vi "Error MSG VicErrorParsing.vi"(11 "WrrmsgIn":string) -> (3 "MsgOut":string[][](array[string]))   [LabVIEW 2019]
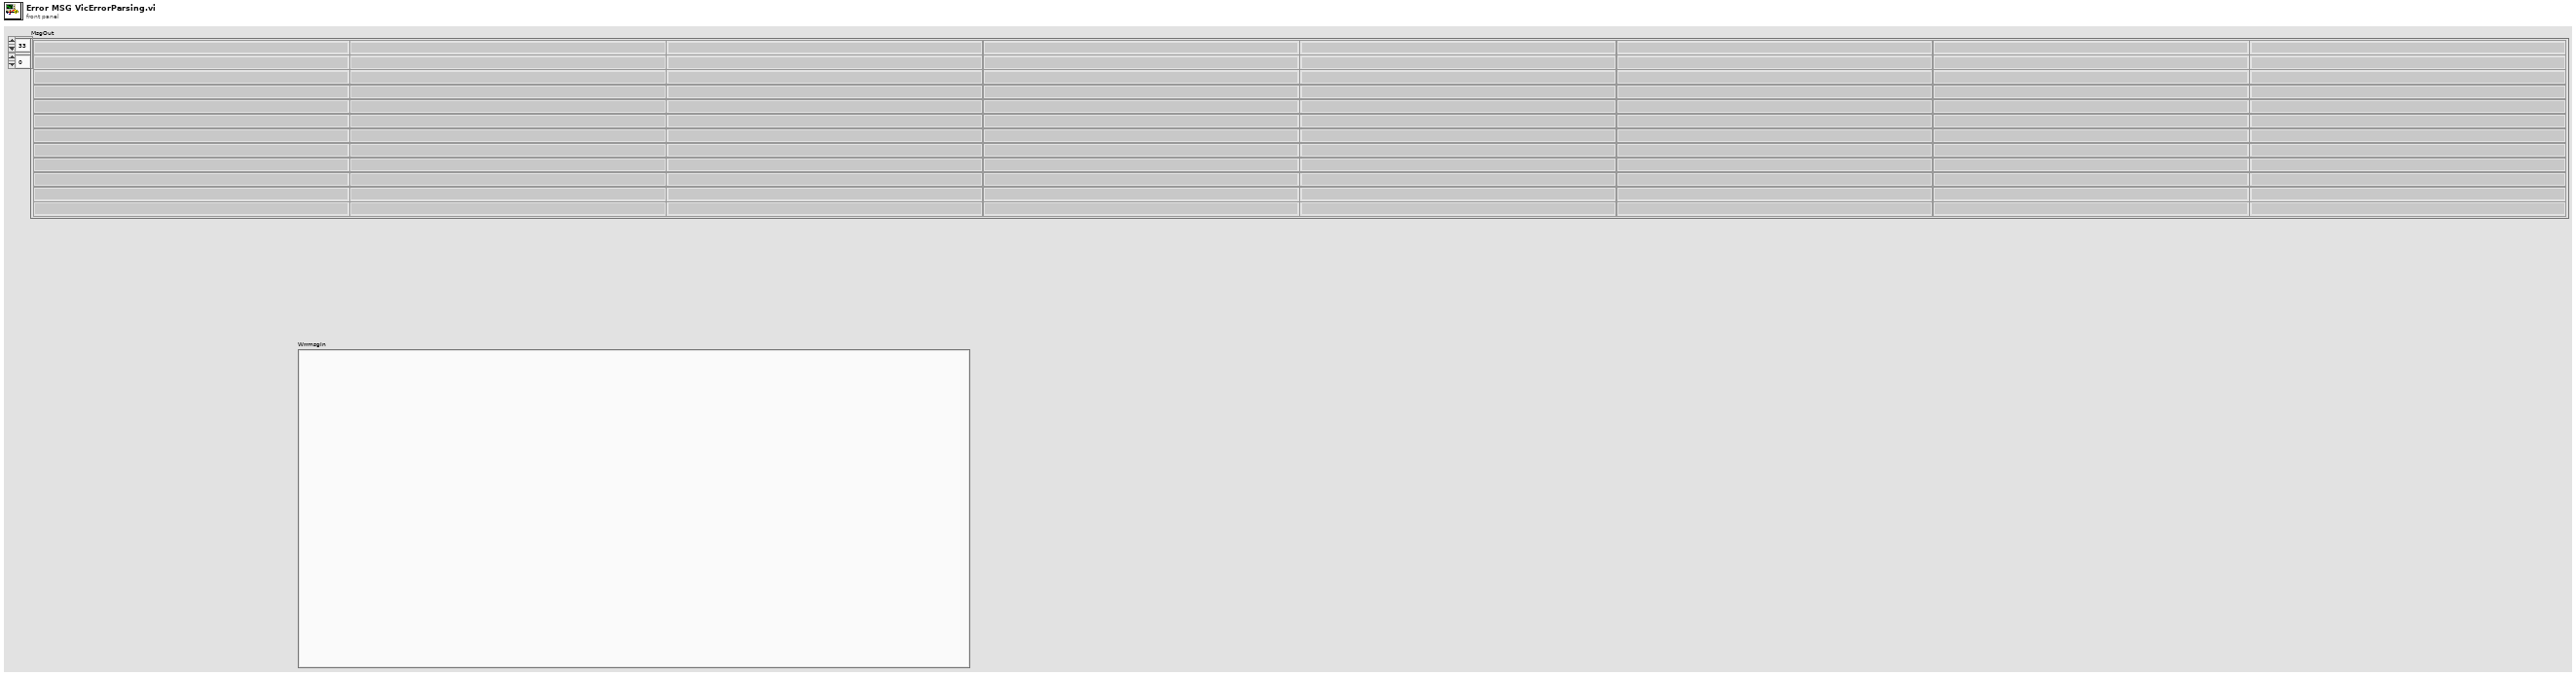
[diagram p1: front panel]
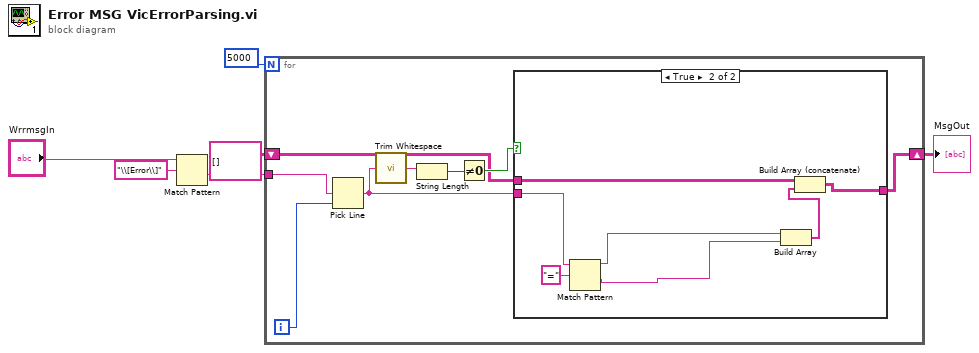
[diagram p0: block diagram]
diagram:
  n1 = Match Pattern(string="WrrmsgIn", regular expression="\\[Error\\]") -> (after substring=w4:string)  [unwired: 1 in, 3 out]
  n2 = for {
    N: 5000 -> [_]
    tunnel: w4 -> [w14]
    shift-right: [w7] -> w1
    shift-left: string[][] [] -> [w9]
    i -> [w13]
    n3 = Pick Line(multi-line string=w14, line index=w13) -> (output string=w8:string)  [unwired: 1 in]
    n4 = call <vilib>:"Trim Whitespace.vi"("string"=w8) -> ("trimmed string"=w12:string)  [unwired: 1 in]
    n5 = String Length(string=w12) -> (length=w11:i32)
    n6 = Not Equal To 0?(x=w11) -> (x != 0?=w10:bool)
    n7 = case shown="True" w10 {
      tunnel: [w15 w22] -> w7
      tunnel: w9 -> [w15 w21]
      tunnel: w8 -> [_ w19]
      frame False {
      }
      frame True {
        n8 = Match Pattern(string=w19, regular expression="=") -> (before substring=w18:string, after substring=w16:string)  [unwired: 1 in, 2 out]
        n9 = Build Array(w18, w16) -> (w17:string[])
        n10 = Build Array (concatenate)(w21, w17) -> (w22:string[][])
      }
    }
  }
  "MsgOut" <- w1
